vi "Do.vi"(8 "error in (no error)":errorcluster, 10 "Actor in":refnum<class "Actor.lvclass">, 11 "Project Number Msg":refnum<class "Project Number Msg.lvclass">) -> (0 "error out":errorcluster, 2 "Actor out":refnum<class "Actor.lvclass">)   [LabVIEW 2013, in "Main View.lvlib" / "Project Number Msg.lvclass"]
doc: "(<B>Filename</B>: Actor Framework.lvlib:Message.lvclass:Do.vi)\n\nDefines what a message does when it is received by an actor. Generally, a message instructs an actor to invoke one of its methods.\n\nBy default, this method does nothing. A child class must override it to define behavior. Create a child class by using the Actor Framework Message Maker dialog box."
uses:
  Project Number Msg.lvclass
  <vilib>/ActorFramework/Actor/Actor.lvclass
  Main View/Main View.lvclass
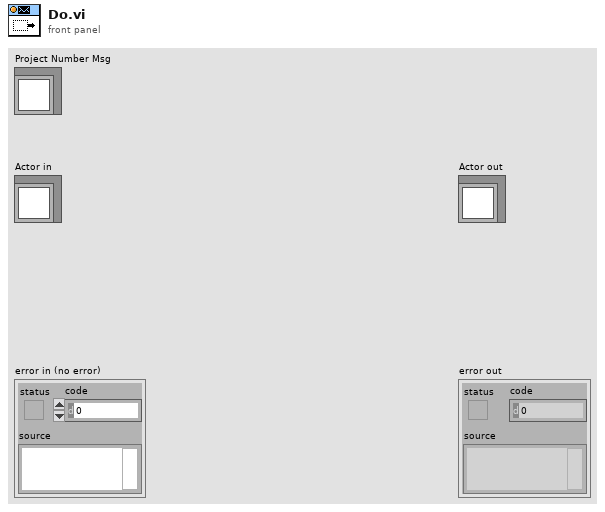
[diagram p1: front panel]
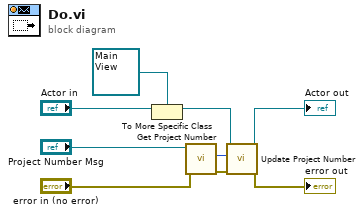
[diagram p0: block diagram]
diagram:
  n1 = To More Specific Class(target class=refnum<class "Main View.lvclass"> refnum ("Main View.lvlib:Main View.lvclass"), reference="Actor in") -> (specific class reference=w5:refnum<class "Main View.lvclass">)  [unwired: 1 in, 1 out]
  n2 = call-dynamic "Get Project Number.vi"("error in (no error)"="error in (no error)", "Project Number Msg in"="Project Number Msg") -> ("error out"=w4:errorcluster, "Project Number"=w6:i32)  [unwired: 7 in, 1 out]
  n3 = call "Update Project Number.vi"("error in (no error)"=w4, "Event Data"=w6, "Main View in"=w5) -> ("error out"=→"error out":errorcluster, "Main View out"=→"Actor out":refnum<class "Main View.lvclass">)  [unwired: 7 in]
